vi "Hardware In - NI 9751-2 (DI Driver).vi"(11 "FPGA Ref":T1) -> ()   [LabVIEW 2015, in "ECS-RT.lvlib"]
uses:
  ECS-RT.lvlib
  Typedefs/FPGA Refs/Generic FPGA Ref.ctl
  <vilib>/Utility/error.llb/Error Cluster From Error Code.vi
  <vilib>/rvi/errors/niLvFpgaAdjustHostInterfaceError.vi
  <vilib>/Powertrain Controls/Device Drivers/Tools/Real-Time/Interp1DTableRT.vi
  <vilib>/rvi/interface/nirviReadWriteControl/nirviReadWriteControl.xnode
  <vilib>/rvi/interface/Simulation/niFpgaSimulationCallBeginRW.vi
  NiFpgaLv.dll
  ECS-Shared.lvlib
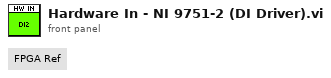
[diagram p1: front panel]
types:
  T1 = typedef "ECS-Shared.lvlib/Generic FPGA Ref.ctl" = refnum<k20>
  T2 = cluster{"ModulePresent":bool, "LVSense":u8, "HVSense":u8, "HVSense2":u8, "TempSense":i8, "Fault1":u8, "Fault2":u8, "OLIntegrator":u32, "HardwareRev":u8, "FirmwareRev":u8}
  T3 = cluster{"FI1OpenCircuit":bool, "FI2OpenCircuit":bool, "FI3OpenCircuit":bool}
  T4 = cluster{"PSCharge":bool, "PSOverLoad":bool, "ShortCircuit":bool, "ModuleTemperature":bool, "HighVoltageDriver":bool, "LowVoltageDriver":bool, "HighVoltageLimit":bool}
  T5 = cluster{"ModulePresent":bool, "Module Temperature (C)":sgl, "Internal High Voltage (V)":sgl, "External High Voltage (V)":sgl, "Battery Voltage (V)":sgl, "Hardware Rev":string, "Firmware Rev":u8}
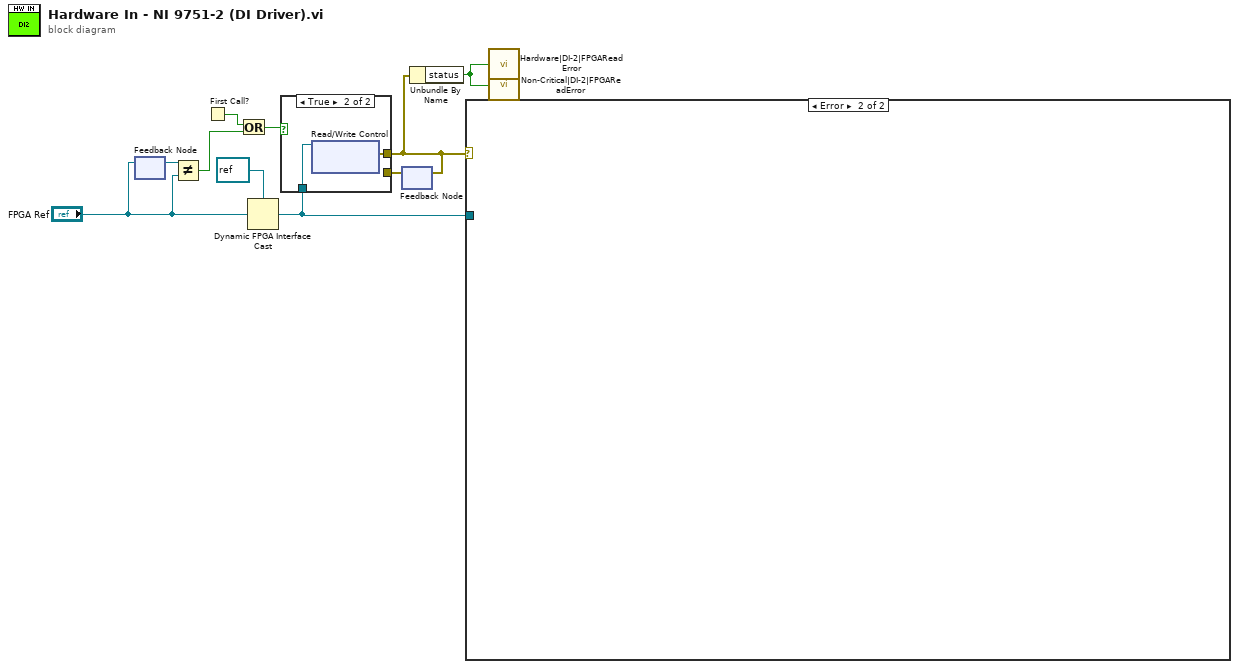
[diagram p0: block diagram]
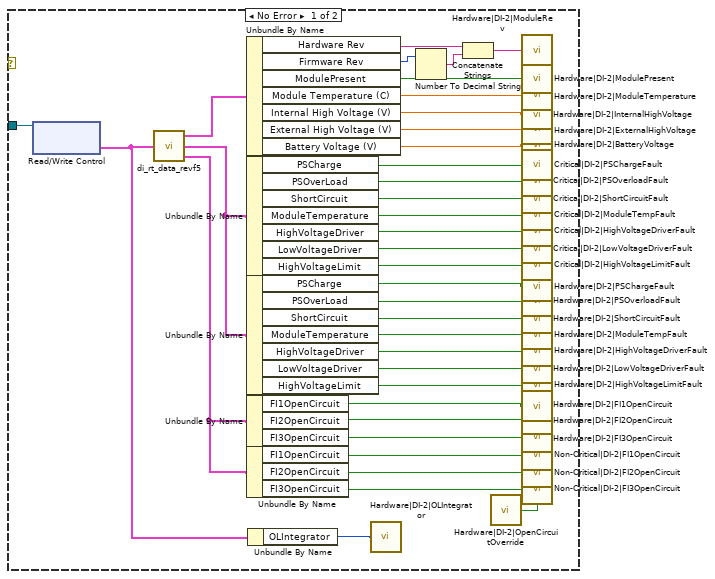
[diagram p3: hidden frame]
diagram:
  n1 = feedback #1() -> (w7:T1)  [unwired: 1 in]
  n2 = feedback-in #1("FPGA Ref") -> ()
  n3 = Not Equal?(x=w7, y="FPGA Ref") -> (x != y?=w6:bool)
  n4 = First Call?() -> (First Call?: T/F=w8:bool)
  n5 = Or(x=w8, y=w6) -> (x .or. y?=w9:bool)
  n6 = Dynamic FPGA Interface Cast(Session In=refnum<k20> refnum ("FPGA VI Reference Out"), Type="FPGA Ref") -> (Session Out=w3:refnum<k20>)
  n7 = feedback #2() -> (w10:errorcluster)  [unwired: 1 in]
  n8 = case shown="True" w9 {
    tunnel: [w11 w13] -> w2
    tunnel: w10 -> [w11 _]
    tunnel: w3 -> [_ w12]
    frame False {
    }
    frame True {
      n9 = xnode "Read/Write Control"("FPGA VI Reference In"=w12) -> ("error out"=w13:errorcluster)  [unwired: 1 in, 2 out]
    }
  }
  n10 = feedback-in #2(w2) -> ()
  n11 = Unbundle By Name(w2) -> ("status"=w1:bool)
  n12 = case shown="Error" w2 {
    tunnel: w3 -> [w14 _]
    frame No Error {
      n13 = xnode "Read/Write Control"("FPGA VI Reference In"=w14) -> ("DI-2.Data"=w45:T2)  [unwired: 1 in, 2 out]
      n14 = call <vilib>:"di_rt_data_revf5.vi"("DIDataFromFPGA"=w45) -> ("Non Critical Faults"=w44:T3, "Critical Faults"=w43:T4, "DIData"=w42:T5)  [unwired: 2 in]
      n15 = Unbundle By Name(w42) -> ("Hardware Rev"=w48:string, "Firmware Rev"=w49:u8, "ModulePresent"=w15:bool, "Module Temperature (C)"=w16:sgl, "Internal High Voltage (V)"=w17:sgl, "External High Voltage (V)"=w18:sgl, "Battery Voltage (V)"=w19:sgl)
      n16 = Unbundle By Name(w43) -> ("PSCharge"=w20:bool, "PSOverLoad"=w21:bool, "ShortCircuit"=w22:bool, "ModuleTemperature"=w23:bool, "HighVoltageDriver"=w24:bool, "LowVoltageDriver"=w25:bool, "HighVoltageLimit"=w26:bool)
      n17 = Unbundle By Name(w43) -> ("PSCharge"=w27:bool, "PSOverLoad"=w28:bool, "ShortCircuit"=w29:bool, "ModuleTemperature"=w30:bool, "HighVoltageDriver"=w31:bool, "LowVoltageDriver"=w32:bool, "HighVoltageLimit"=w33:bool)
      n18 = Unbundle By Name(w44) -> ("FI1OpenCircuit"=w34:bool, "FI2OpenCircuit"=w35:bool, "FI3OpenCircuit"=w36:bool)
      n19 = Unbundle By Name(w44) -> ("FI1OpenCircuit"=w37:bool, "FI2OpenCircuit"=w38:bool, "FI3OpenCircuit"=w39:bool)
      n20 = Unbundle By Name(w45) -> ("OLIntegrator"=w41:u32)
      n21 = call "Hardware|DI-2|OLIntegrator"("Value"=w41) -> ()
      n22 = Number To Decimal String(number=w49) -> (decimal integer string=w47:string)  [unwired: 1 in]
      n23 = Concatenate Strings(w48, w47) -> (w46:string)
      n24 = call "Hardware|DI-2|OpenCircuitOverride"() -> ("Value"=w40:bool)
      n25 = call "Hardware|DI-2|ModuleRev"("Value"=w46) -> ()
      n26 = call "Hardware|DI-2|ModulePresent"("Value"=w15) -> ()
      n27 = call "Hardware|DI-2|ModuleTemperature"("Value"=w16) -> ()
      n28 = call "Hardware|DI-2|InternalHighVoltage"("Value"=w17) -> ()
      n29 = call "Hardware|DI-2|ExternalHighVoltage"("Value"=w18) -> ()
      n30 = call "Hardware|DI-2|BatteryVoltage"("Value"=w19) -> ()
      n31 = call "Critical|DI-2|PSChargeFault"("Fault"=w20) -> ()  [unwired: 2 in]
      n32 = call "Critical|DI-2|PSOverloadFault"("Fault"=w21) -> ()  [unwired: 2 in]
      n33 = call "Critical|DI-2|ShortCircuitFault"("Fault"=w22) -> ()  [unwired: 2 in]
      n34 = call "Critical|DI-2|ModuleTempFault"("Fault"=w23) -> ()  [unwired: 2 in]
      n35 = call "Critical|DI-2|HighVoltageDriverFault"("Fault"=w24) -> ()  [unwired: 2 in]
      n36 = call "Critical|DI-2|LowVoltageDriverFault"("Fault"=w25) -> ()  [unwired: 2 in]
      n37 = call "Critical|DI-2|HighVoltageLimitFault"("Fault"=w26) -> ()  [unwired: 2 in]
      n38 = call "Hardware|DI-2|PSChargeFault"("Value"=w27) -> ()
      n39 = call "Hardware|DI-2|PSOverloadFault"("Value"=w28) -> ()
      n40 = call "Hardware|DI-2|ShortCircuitFault"("Value"=w29) -> ()
      n41 = call "Hardware|DI-2|ModuleTempFault"("Value"=w30) -> ()
      n42 = call "Hardware|DI-2|HighVoltageDriverFault"("Value"=w31) -> ()
      n43 = call "Hardware|DI-2|LowVoltageDriverFault"("Value"=w32) -> ()
      n44 = call "Hardware|DI-2|HighVoltageLimitFault"("Value"=w33) -> ()
      n45 = call "Hardware|DI-2|FI1OpenCircuit"("Value"=w34) -> ()
      n46 = call "Hardware|DI-2|FI2OpenCircuit"("Value"=w35) -> ()
      n47 = call "Hardware|DI-2|FI3OpenCircuit"("Value"=w36) -> ()
      n48 = call "Non-Critical|DI-2|FI1OpenCircuit"("Fault"=w37, "Override (F)"=w40) -> ()  [unwired: 1 in]
      n49 = call "Non-Critical|DI-2|FI2OpenCircuit"("Fault"=w38, "Override (F)"=w40) -> ()  [unwired: 1 in]
      n50 = call "Non-Critical|DI-2|FI3OpenCircuit"("Fault"=w39, "Override (F)"=w40) -> ()  [unwired: 1 in]
    }
    frame Error {
    }
  }
  n51 = call "Hardware|DI-2|FPGAReadError"("Value"=w1) -> ()
  n52 = call "Non-Critical|DI-2|FPGAReadError"("Fault"=w1) -> ()  [unwired: 2 in]
